vi "ReadHeader.vi"(8 "error in (no error)":errorcluster, 11 "Byte Stream File in":refnum<file>) -> (0 "error out":errorcluster, 1 "Number of tracks":u16, 2 "Format":u16, 3 "Byte Stream File out":refnum<file>, 5 "Division":u16)   [LabVIEW 2016]
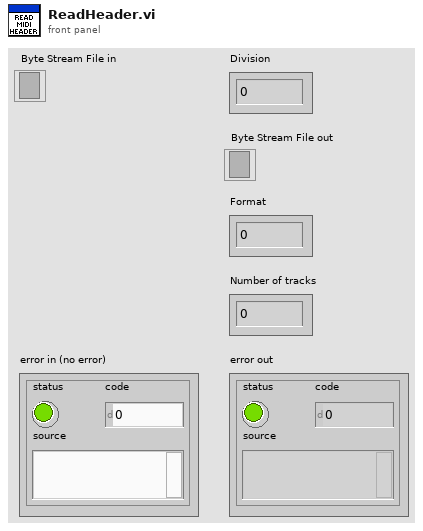
[diagram p1: front panel]
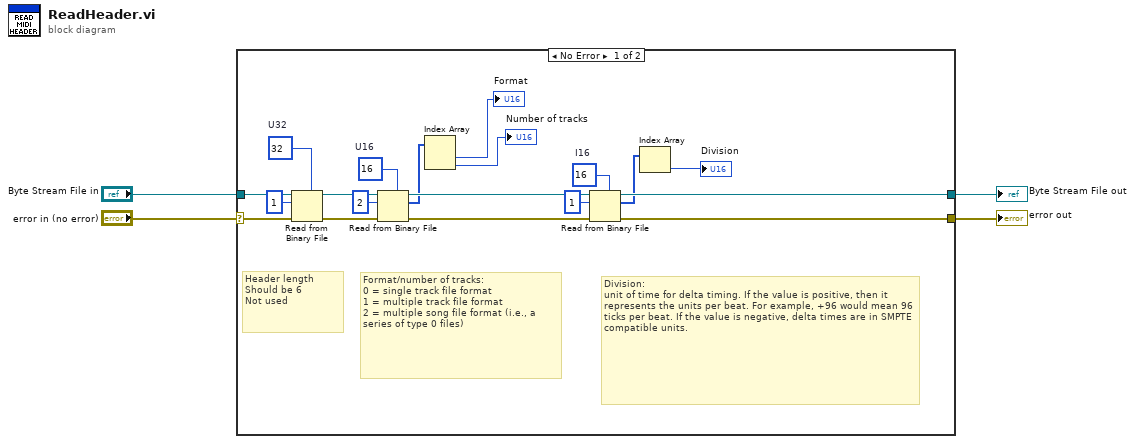
[diagram p0: block diagram]
diagram:
  n1 = case shown="No Error" "error in (no error)" {
    selector: "error in (no error)" -> [w5 w25]
    tunnel: [w23 w25] -> w4
    tunnel: [w22 w24] -> w3
    tunnel: "Byte Stream File in" -> [w6 w24]
    frame No Error {
      w19 = u16 16  # I16
      w12 = u16 16  # U16
      w8 = u32 32  # U32
      # "Division:\nunit of time for delta timing. If the value is positive, then it represents the units per beat. For example, +96 would mean 96 ticks per beat. If the value is negative, delta times are in SMPTE compatible units."
      # "Format/number of tracks:\n0 = single track file format \n1 = multiple track file format \n2 = multiple song file format (i.e., a series of type 0 files)"
      # "Header length\nShould be 6\nNot used"
      n2 = Read from Binary File(5:w8, 8:w5, 10:1 ("count (1)"), 11:w6) -> (0:w10:errorcluster, 3:w9:refnum<file>)  [unwired: 2 in, 2 out]
      n3 = Read from Binary File(5:w12, 8:w10, 10:2 ("count (1)"), 11:w9) -> (0:w17:errorcluster, 2:w13:u16[], 3:w16:refnum<file>)  [unwired: 2 in, 1 out]
      n4 = Index Array(array=w13) -> (element #1=→"Format":u16, element #2=→"Number of tracks":u16)  [unwired: 2 in]
      n5 = Read from Binary File(5:w19, 8:w17, 10:1 ("count (1)"), 11:w16) -> (0:w23:errorcluster, 2:w20:u16[], 3:w22:refnum<file>)  [unwired: 2 in, 1 out]
      n6 = Index Array(array=w20) -> (element=→"Division":u16)  [unwired: 1 in]
    }
    frame Error {
    }
  }
  "error out" <- w4
  "Byte Stream File out" <- w3
